vi "confirmerCommande.vi"(1 "num_cmd":string, 2 "?":bool) -> ()   [LabVIEW 2024]
uses:
  <vilib>/drjdpowell/SQLite Library/SQL Connection/Open (string).vi
  <vilib>/drjdpowell/SQLite Library/SQL Connection/Execute SQL.vi
  <vilib>/drjdpowell/SQLite Library/SQL Connection/Connection.lvclass
  <vilib>/drjdpowell/SQLite Library/SQLite.lvlib
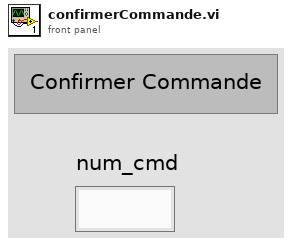
[diagram p1: front panel]
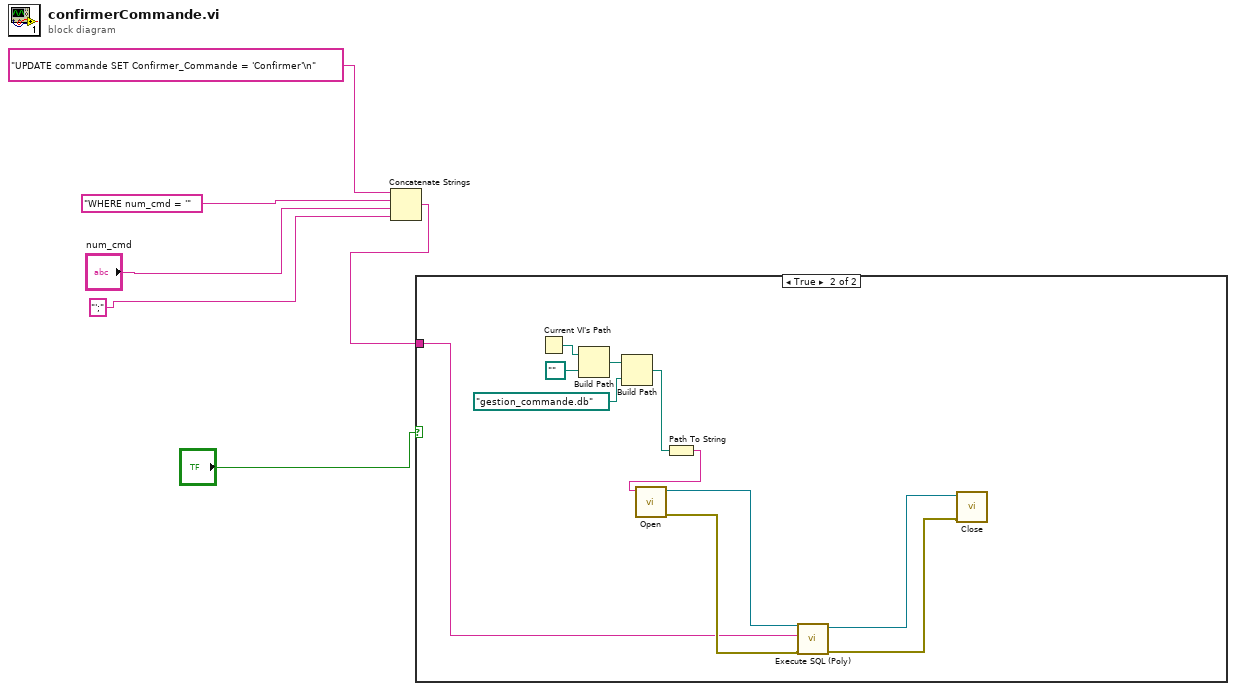
[diagram p0: block diagram]
diagram:
  n1 = Concatenate Strings("UPDATE commande SET Confirmer_Commande = 'Confirmer'\n", "WHERE num_cmd = '", "num_cmd", "';") -> (w1:string)
  n2 = case shown="True" "?" {
    tunnel: w1 -> [_ w13]
    frame False {
    }
    frame True {
      n3 = Current VI's Path() -> (path=w12:path)
      n4 = Build Path(base path=w12, name or relative path=path "..") -> (appended path=w9:path)
      n5 = Build Path(base path=w9, name or relative path=path "gestion_commande.db" ("Filename")) -> (appended path=w8:path)
      n6 = Path To String(path=w8) -> (string=w7:string)
      n7 = call-poly <vilib>:"Open.vi"("db file"=w7) -> ("error out"=w17:errorcluster, "SQLite Connection"=w14:refnum<class "Connection.lvclass">)  [unwired: 9 in]
      n8 = call-poly <vilib>:"Execute SQL (Poly).vi"("error in (no error)"=w17, "SQL"=w13, "SQLite Connection in"=w14) -> ("error out"=w16:errorcluster, "SQLite Connection"=w15:refnum<class "Connection.lvclass">)  [unwired: 5 in, 2 out]
      n9 = call-dynamic "Close.vi"("error in (no error)"=w16, "SQLite Connection in"=w15) -> ()  [unwired: 9 in, 1 out]
    }
  }
